vi "encode_data.vi"(7 "data type":enum16{"U16", "I32"}(ring), 8 "error in (no error)":errorcluster, 10 "data I32":i32, 11 "DL090602SutterMP285Stage in":refnum<class "StageMMS2015ASI.lvclass">) -> (0 "error out":errorcluster, 2 "encoded data":string, 3 "DL090602SutterMP285Stage out":refnum<class "StageMMS2015ASI.lvclass">)   [LabVIEW 2010, in "StageMMS2015ASI.lvclass"]
uses:
  StageMMS2015ASI.lvclass
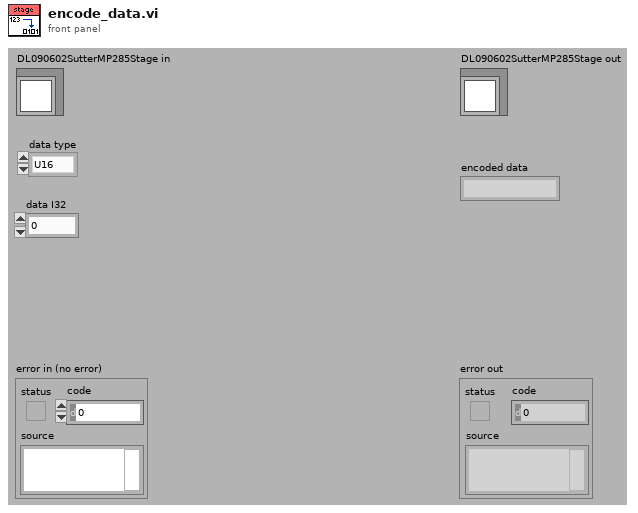
[diagram p1: front panel]
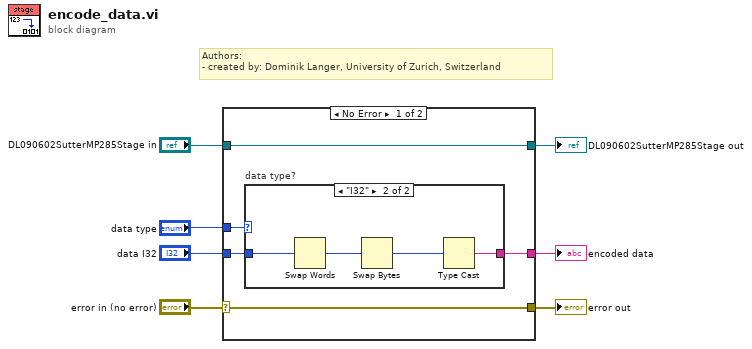
[diagram p0: block diagram]
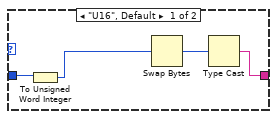
[diagram p2: hidden frame]
diagram:
  # "Authors: \n- created by: Dominik Langer, University of Zurich, Switzerland"
  n1 = case shown="No Error" "error in (no error)" {
    selector: "error in (no error)" -> [w11 w22]
    tunnel: [w11 w22] -> w6
    tunnel: [w12 w21] -> w4
    tunnel: "DL090602SutterMP285Stage in" -> [w12 w21]
    tunnel: "data type" -> [w10 _]
    tunnel: "data I32" -> [w9 _]
    tunnel: [w8 _] -> w1
    frame No Error {
      n2 = case "data type?" shown="\"I32\"" w10 {
        tunnel: [w16 w18] -> w8
        tunnel: w9 -> [w14 w17]
        frame "U16", Default {
          n3 = To Unsigned Word Integer(number=w14) -> (unsigned 16bit integer=w13:u16)
          n4 = Swap Bytes(anything=w13) -> (byte swapped=w15:u16)
          n5 = Type Cast(x=w15) -> (*(type *) &x=w16:string)  [unwired: 1 out]
        }
        frame "I32" {
          n6 = Swap Words(1:w17) -> (0:w19:i32)
          n7 = Swap Bytes(anything=w19) -> (byte swapped=w20:i32)
          n8 = Type Cast(x=w20) -> (*(type *) &x=w18:string)  [unwired: 1 out]
        }
      }
    }
    frame Error {
    }
  }
  "error out" <- w6
  "DL090602SutterMP285Stage out" <- w4
  "encoded data" <- w1
